vi "NIMS_NS_fir_lpnorm.vi"(5 "Function name":string, 6 "Line number":i32, 7 "Number of outputs requested":i32, 8 "error in (no error)":errorcluster, 11 "[A]":variant[](array[variant])) -> (0 "error out":errorcluster, 3 "[funct(A)]":variant[](array[variant]))   [LabVIEW 2017]
uses:
  <vilib>/imath/engines/lvmath/Functions/Error Handling/error.ctl
  <instcachedir>/0/NIMS_RunTimeType_From StrictType (excl LVString)_1019F277F0A747EDBCA0F6C52CA54500.lvgen/NIMS_RunTimeType_From StrictType (excl LVString)_1019F277F0A747EDBCA0F6C52CA54500_000.vi
  <instcachedir>/0/NIMS_Get Scalar_w Error_1987D997E87247DDAC16EA23A5E9E4FC.lvgen/NIMS_Get Scalar_w Error_1987D997E87247DDAC16EA23A5E9E4FC_000.vi
  <instcachedir>/0/NIMS_Complex To Real_BE01396FDE034E8E94CEBBA1E368668D.lvgen/NIMS_Complex To Real_BE01396FDE034E8E94CEBBA1E368668D_000.vi
  <instcachedir>/0/NIMS_Get Any Vector_w Error - Matrix_9FDB8FBE264C42EDBC8FF9BA66C3EF33.lvgen/NIMS_Get Any Vector_w Error - Matrix_9FDB8FBE264C42EDBC8FF9BA66C3EF33_001.vi
  <instcachedir>/0/NIMS_RunTimeType_To Numeric_1CBDAFC4EFAD4045A1DE52278D16738D.lvgen/NIMS_RunTimeType_To Numeric_1CBDAFC4EFAD4045A1DE52278D16738D_000.vi
  <vilib>/addons/Digital Filter Design/NI_DigFilter_MathScript.lvlib
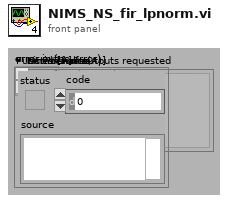
[diagram p1: front panel]
types:
  T1 = typedef "error.ctl" = enum16{"No Error", "Problem", "Input type must not be void", "Incorrect number of parameters", "Function not defined for non-numeric types", "An output variable of the user-defined function is undefined", "Function only defined for character arrays", "Function not defined for boolean, character, or single precision", "Function not defined for complex types", "Not a valid operation", "Inputs must be scalar", "Input matrices are not the same size", "Function only available on RT", "Input matrices must be nonnegative integers of the same type", "Arguments must be non-negative integers less than bitmax", "Number to complement must be less than 2^N", "Bit to get is outside range", "Bit to set is outside range", "Input must be real type ", "At least one parameter must be scalar", "Unable to display plug-in data on RT", "Function not defined for higher dimensional matrices", "Invalid attributes", "Wrong Type of Input Arguments", "Wrong Argument Option", "Invalid file identifier", "Indices must be real positive integers", "The variable is not a matrix data type.", "Number of elements must be the same for indices and values", "You cannot replace elements of a matrix with non-matrix data types.", "Cannot resize a 2D matrix with a linear index", "Unknown variable or symbol", "Indices out of range", "Empty matrix deletion can not be used with two indices", "Number of rows and columns must be the same for indices and values.", "Complex cannot be converted to Boolean", "Char cannot be converted to Boolean", "int64 cannot be converted to Boolean", "uint64 cannot be converted to Boolean", "You cannot convert a Boolean to a character.", "Incompatible input size in 3D surface function", "All rows must have the same number of columns", "Incompatible types", "Invalid matrix dimensions", "Dimension must be 1 or 2", "Base must be an integer between 2 and 36", "Invalid input", "Square matrix required", "Function 'timerstart' must be called before 'timerstop'", "Arguments must be positive real", "Step must not be zero", "Wrong number of input arguments", "Wrong number of output arguments", "Too many index arguments", "Input scalar must be >= 0", "Input scalar must be positive", "Input scalar must not be 0", "Input scalar must be in range [0,1]", "Can't use conditionally defined variable that's undefined", "Input must be a vector", "RT Exec Trace Toolkit not licensed", "Empty vector error", "All elements must be in domain [-1,1]", "All real elements of input vector must be >= 0", "All elements of input vector must be positive", "Values of input vectors are not compatible", "DAQmx not installed", "Input vector must be an increasing vector", "Dereferenced field does not exist within the struct", "A vector or matrix of structures must be indexed before it can be dereferenced", "Lenths of two input vectors are not compatible", "Invalid fieldname", "Empty matrix error", "Cannot use '.' on a type other than Struct", "Unused074", "Data type of the struct's field name is invalid", "Using . to dereference data that is not a struct", "Input struct contains invalid type ", "Size of input matrix is incompatible with input size", "Invalid format specifier", "Could not find field within struct", "Bad permutation array", "Mismatched fieldnames", "ode: User Function could not be opened", "ode: User Function signature does not meet ode requirements", "Unused085", "RunTime: MathScript could not be compiled", "Unknown function", "Only scalars and strings supported", "ode: User Function signature has incorrect number of inputs", "ode:User Function signature has incorrect number of outputs", "Range is too large", "End used without variable", "Function not available (RTE)", "Custom user error", "Arguments must be integers less than bitmax", "Shared library not found", "Header file not found", "Shared library already loaded", "Shared library not loaded", "Shared library function not found", "Shared library string return problem", "Problem calling shared library function", "Problem loading shared library from OS", "Problem parsing shared library header file", "Shared library incompatible types", "Shared library unsupported return type", "Shared library function not exported", "Shared library unsupported input type", "Problem unloading shared library from OS", "Function only available from UI", "Function specified in argument is missing", "An internal error has occurred", "Invalid object", "Invalid property", "Read-only property", "A break command has occurred", "A continue command has occurred", "A return command has occurred", "ode: times parameter invalid", "Function specified in argument has incorrect signature", "Function not found in file", "Reserved keyword cannot be defined as variable", "Reserved keyword cannot be defined as a function or script", "Arguments must be string literals", "Function not supported on this platform", "All columns must have the same number of rows", "Function ignored in RTE warning", "Cannot use : as a parameter that is not a variable", "Output can't be coerced to requested type", "Function not supported on current target", "Variable dependent on an unwired function input", "Unused132", "Unused133", "Unused134", "Unused135", "Unused136", "Unused137", "Unused138", "Unused139", "Global/Persistent must only take constants as arguments.", "Varargin must be last input in the function definition.", "Varargout must be last output in the function definition.", "Invalid output type. Cannot output a cell array of any type other than string.", "Invalid output type. Type is a dynamic struct.", "Invalid output type. Type is a struct that has a field whose type is not known until run-time", "Invalid output type. Type is a struct that has a field which is a plot object.", "MathScript parser DLL missing", "MathScript requires LabVIEW Full", "MathScript license is invalid or missing", "Varargout not supported except in assignments."}
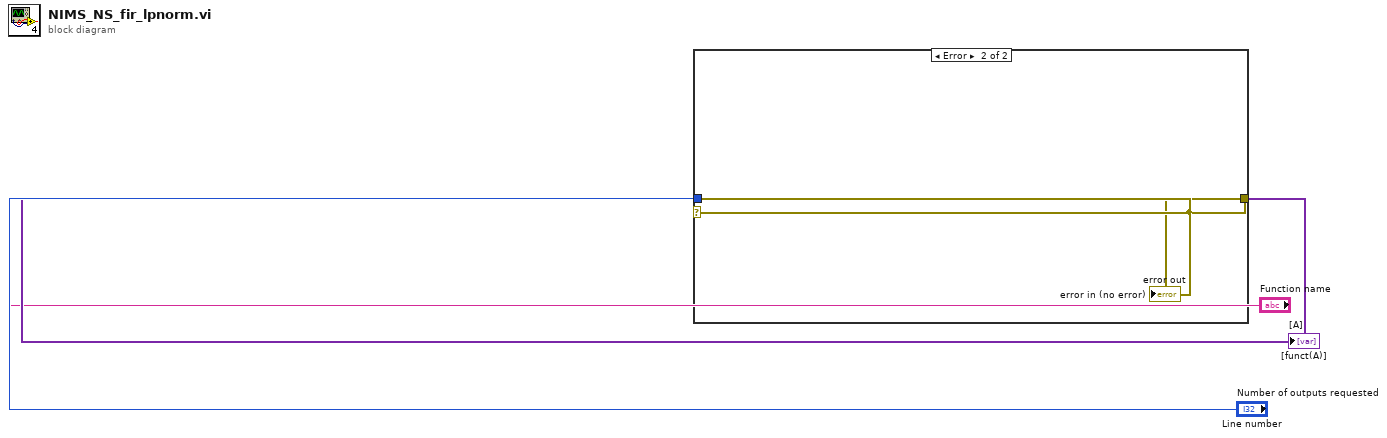
[diagram p0: block diagram]
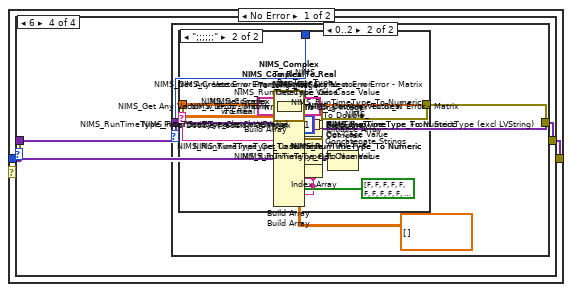
[diagram p2: hidden frame]
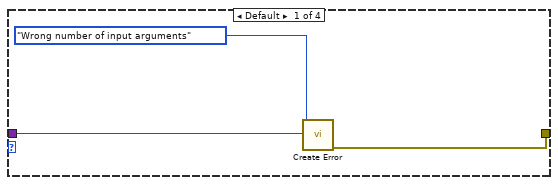
[diagram p3: hidden frame]
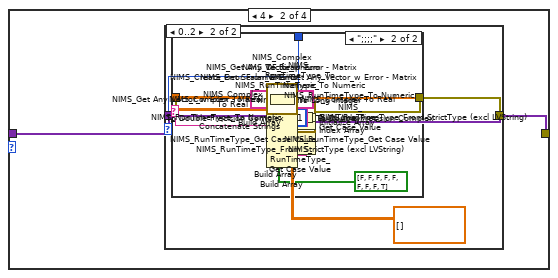
[diagram p4: hidden frame]
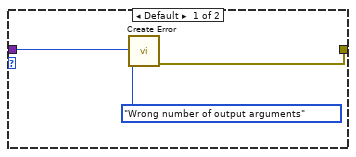
[diagram p5: hidden frame]
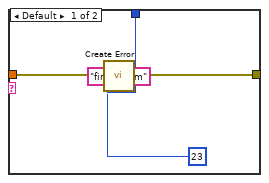
[diagram p6: hidden frame]
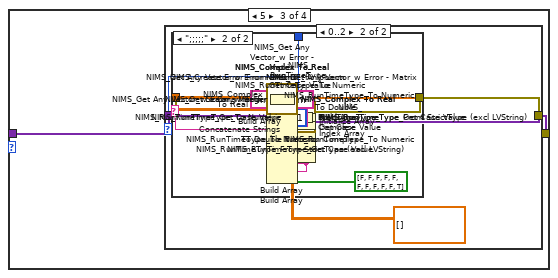
[diagram p7: hidden frame]
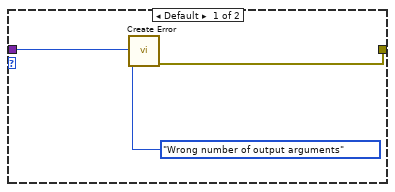
[diagram p8: hidden frame]
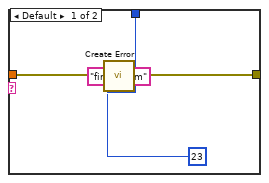
[diagram p9: hidden frame]
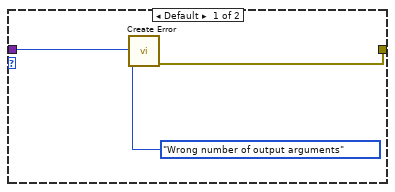
[diagram p10: hidden frame]
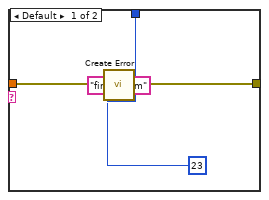
[diagram p11: hidden frame]
diagram:
  n1 = case shown="Error" "error in (no error)" {
    selector: "error in (no error)" -> [_ w295]
    tunnel: [w15 _] -> w4
    tunnel: [w14 w295] -> w3
    tunnel: "error in (no error)" -> [w13 _]
    tunnel: "Number of outputs requested" -> [w12 _]
    tunnel: "[A]" -> [w11 _]
    tunnel: "Function name" -> [w10 _]
    tunnel: "Line number" -> [w9 _]
    frame No Error {
      n2 = Array Size(array=w11) -> (size(s)=w8:i32)
      n3 = case shown="6" w8 {
        tunnel: [_ w27 w109 w200] -> w15
        tunnel: w10 -> [w19 w24 w106 w197]
        tunnel: w9 -> [w20 w25 w107 w198]
        tunnel: w13 -> [w17 w23 w105 w196]
        tunnel: [w16 w22 w104 w195] -> w14
        tunnel: w12 -> [_ w21 w103 w194]
        tunnel: w11 -> [_ w26 w108 w199]
        frame Default {
          n4 = call <vilib>:"Create Error.vi"("Function name"=w19, "error in (no error)"=w17, "Error Enum"=error."Wrong number of input arguments", "Line number"=w20) -> ("error out"=w16:errorcluster)  [unwired: 6 in, 1 out]
        }
        frame 4 {
          n5 = case shown="0..2" w21 {
            tunnel: [_ w33] -> w27
            tunnel: w24 -> [w31 _]
            tunnel: w25 -> [w32 w64]
            tunnel: w23 -> [w29 w62]
            tunnel: [w28 w45] -> w22
            tunnel: w26 -> [_ w65]
            frame Default {
              n6 = call <vilib>:"Create Error.vi"("Function name"=w31, "error in (no error)"=w29, "Error Enum"=error."Wrong number of output arguments", "Line number"=w32) -> ("error out"=w28:errorcluster)  [unwired: 6 in, 1 out]
            }
            frame 0..2 {
              w39 = 1
              n7 = Index Array(array=w65) -> (element #1=w61:variant, element #2=w57:variant, element #3=w53:variant, element #4=w49:variant)  [unwired: 4 in]
              n8 = call <vilib>:"NIMS_RunTimeType_Get Case Value.vi"("Data In"=w49) -> ("Case Value"=w46:string)  [unwired: 9 in, 1 out]
              n9 = call-generic <vilib>:"NIMS_RunTimeType_To Numeric.vi"("DataType"=cdb[][] [], "Variant"=w49) -> ("data"=w47:cdb[][])  [unwired: 1 in]
              n10 = call <vilib>:"NIMS_RunTimeType_Get Case Value.vi"("Data In"=w53) -> ("Case Value"=w50:string)  [unwired: 9 in, 1 out]
              n11 = call-generic <vilib>:"NIMS_RunTimeType_To Numeric.vi"("DataType"=cdb[][] [], "Variant"=w53) -> ("data"=w51:cdb[][])  [unwired: 1 in]
              n12 = call <vilib>:"NIMS_RunTimeType_Get Case Value.vi"("Data In"=w57) -> ("Case Value"=w54:string)  [unwired: 9 in, 1 out]
              n13 = call-generic <vilib>:"NIMS_RunTimeType_To Numeric.vi"("DataType"=cdb[][] [], "Variant"=w57) -> ("data"=w55:cdb[][])  [unwired: 1 in]
              n14 = call <vilib>:"NIMS_RunTimeType_Get Case Value.vi"("Data In"=w61) -> ("Case Value"=w58:string)  [unwired: 9 in, 1 out]
              n15 = call-generic <vilib>:"NIMS_RunTimeType_To Numeric.vi"("DataType"=cdb[][] [], "Variant"=w61) -> ("data"=w59:cdb[][])  [unwired: 1 in]
              n16 = Concatenate Strings(w58, w54, w50, w46) -> (w63:string)
              n17 = case shown="\";;;;\"" w63 {
                tunnel: w62 -> [w67 w77]
                tunnel: [_ w72] -> w44
                tunnel: [_ w71] -> w40
                tunnel: [w66 w73] -> w45
                tunnel: w59 -> [_ w101]
                tunnel: w55 -> [_ w97]
                tunnel: w51 -> [_ w94]
                tunnel: w47 -> [_ w91]
                tunnel: w64 -> [w70 w80]
                frame Default {
                  n18 = call <vilib>:"Create Error.vi"("Function name"="fir_lpnorm", "error in (no error)"=w67, "Error Enum"=23, "Line number"=w70) -> ("error out"=w66:errorcluster)  [unwired: 6 in, 1 out]
                }
                frame ";;;;" {
                  w75 = "fir_lpnorm"
                  n19 = call-generic <vilib>:"NIMS_Complex To Real.vi"("A"=w91) -> ("Error Enum"=w83:T1, "Real(A)"=w90:dbl[][])  [unwired: 8 in, 1 out]
                  n20 = call-generic <vilib>:"NIMS_Get Any Vector_w Error - Matrix.vi"("A"=w90) -> ("Error Enum"=w82:T1, "Vector"=w92:dbl[])  [unwired: 8 in, 1 out]
                  n21 = call-generic <vilib>:"NIMS_Complex To Real.vi"("A"=w94) -> ("Error Enum"=w85:T1, "Real(A)"=w93:dbl[][])  [unwired: 8 in, 1 out]
                  n22 = call-generic <vilib>:"NIMS_Get Any Vector_w Error - Matrix.vi"("A"=w93) -> ("Error Enum"=w84:T1, "Vector"=w95:dbl[])  [unwired: 8 in, 1 out]
                  n23 = call-generic <vilib>:"NIMS_Complex To Real.vi"("A"=w97) -> ("Error Enum"=w87:T1, "Real(A)"=w96:dbl[][])  [unwired: 8 in, 1 out]
                  n24 = call-generic <vilib>:"NIMS_Get Any Vector_w Error - Matrix.vi"("A"=w96) -> ("Error Enum"=w86:T1, "Vector"=w98:dbl[])  [unwired: 8 in, 1 out]
                  n25 = call-generic <vilib>:"NIMS_Complex To Real.vi"("A"=w101) -> ("Error Enum"=w89:T1, "Real(A)"=w100:dbl[][])  [unwired: 8 in, 1 out]
                  n26 = To Long Integer(number=w100) -> (32bit integer=w99:i32[][])
                  n27 = call-generic <vilib>:"NIMS_Get Scalar_w Error.vi"("A"=w99) -> ("Error Enum"=w88:T1, "Scalar"=w102:i32)  [unwired: 8 in, 1 out]
                  n28 = call <vilib>:"NIMS_DF_fir_lpnorm.vi"("mag"=w92, "e"=w95, "f"=w98, "n"=w102) -> ("error"=w81:i32, "err"=w71:dbl, "b"=w72:dbl[])  [unwired: 5 in]
                  n29 = Build Array(w75, w75, w75, w75, w75, w75, w75, w75, "fir_lpnorm") -> (w78:string[])
                  n30 = Build Array(w89, w88, w87, w86, w85, w84, w83, w82, w81) -> (w79:i32[])
                  n31 = call <vilib>:"NIMS_Create Error From Enums.vi"("Error Code"=bool[] [FALSE, FALSE, FALSE, FALSE, FALSE, FALSE, FALSE, FALSE, TRUE], "error in (no error)"=w77, "Line no"=w80, "Error Enums"=w79, "Function names"=w78) -> ("error out"=w73:errorcluster)  [unwired: 6 in]
                }
              }
              n32 = Initialize Array(w40, w39, w39) -> (w38:dbl[][])
              n33 = To Double Precision Complex(1:w38) -> (0:w37:cdb[][])
              n34 = call-generic <vilib>:"NIMS_RunTimeType_From StrictType (excl LVString).vi"("Plug-In Name"="", "Data In"=w37) -> ("Data Out"=w34:variant)  [unwired: 2 in]
              n35 = Build Array(w44) -> (w43:dbl[][])
              n36 = To Double Precision Complex(1:w43) -> (0:w42:cdb[][])
              n37 = call-generic <vilib>:"NIMS_RunTimeType_From StrictType (excl LVString).vi"("Plug-In Name"="", "Data In"=w42) -> ("Data Out"=w35:variant)  [unwired: 2 in]
              n38 = Build Array(w35, w34) -> (w33:variant[])
            }
          }
        }
        frame 5 {
          n39 = case shown="0..2" w103 {
            tunnel: [_ w115] -> w109
            tunnel: w106 -> [w113 _]
            tunnel: w107 -> [w114 w150]
            tunnel: w105 -> [w111 w148]
            tunnel: [w110 w127] -> w104
            tunnel: w108 -> [_ w151]
            frame Default {
              n40 = call <vilib>:"Create Error.vi"("Function name"=w113, "error in (no error)"=w111, "Error Enum"=error."Wrong number of output arguments", "Line number"=w114) -> ("error out"=w110:errorcluster)  [unwired: 6 in, 1 out]
            }
            frame 0..2 {
              w121 = 1
              n41 = Index Array(array=w151) -> (element #1=w147:variant, element #2=w143:variant, element #3=w139:variant, element #4=w135:variant, element #5=w131:variant)  [unwired: 5 in]
              n42 = call <vilib>:"NIMS_RunTimeType_Get Case Value.vi"("Data In"=w131) -> ("Case Value"=w128:string)  [unwired: 9 in, 1 out]
              n43 = call-generic <vilib>:"NIMS_RunTimeType_To Numeric.vi"("DataType"=cdb[][] [], "Variant"=w131) -> ("data"=w129:cdb[][])  [unwired: 1 in]
              n44 = call <vilib>:"NIMS_RunTimeType_Get Case Value.vi"("Data In"=w135) -> ("Case Value"=w132:string)  [unwired: 9 in, 1 out]
              n45 = call-generic <vilib>:"NIMS_RunTimeType_To Numeric.vi"("DataType"=cdb[][] [], "Variant"=w135) -> ("data"=w133:cdb[][])  [unwired: 1 in]
              n46 = call <vilib>:"NIMS_RunTimeType_Get Case Value.vi"("Data In"=w139) -> ("Case Value"=w136:string)  [unwired: 9 in, 1 out]
              n47 = call-generic <vilib>:"NIMS_RunTimeType_To Numeric.vi"("DataType"=cdb[][] [], "Variant"=w139) -> ("data"=w137:cdb[][])  [unwired: 1 in]
              n48 = call <vilib>:"NIMS_RunTimeType_Get Case Value.vi"("Data In"=w143) -> ("Case Value"=w140:string)  [unwired: 9 in, 1 out]
              n49 = call-generic <vilib>:"NIMS_RunTimeType_To Numeric.vi"("DataType"=cdb[][] [], "Variant"=w143) -> ("data"=w141:cdb[][])  [unwired: 1 in]
              n50 = call <vilib>:"NIMS_RunTimeType_Get Case Value.vi"("Data In"=w147) -> ("Case Value"=w144:string)  [unwired: 9 in, 1 out]
              n51 = call-generic <vilib>:"NIMS_RunTimeType_To Numeric.vi"("DataType"=cdb[][] [], "Variant"=w147) -> ("data"=w145:cdb[][])  [unwired: 1 in]
              n52 = Concatenate Strings(w144, w140, w136, w132, w128) -> (w149:string)
              n53 = case shown="\";;;;;\"" w149 {
                tunnel: w148 -> [w153 w163]
                tunnel: [_ w158] -> w126
                tunnel: [_ w157] -> w122
                tunnel: [w152 w159] -> w127
                tunnel: w145 -> [_ w192]
                tunnel: w141 -> [_ w188]
                tunnel: w137 -> [_ w185]
                tunnel: w133 -> [_ w182]
                tunnel: w129 -> [_ w179]
                tunnel: w150 -> [w156 w166]
                frame Default {
                  n54 = call <vilib>:"Create Error.vi"("Function name"="fir_lpnorm", "error in (no error)"=w153, "Error Enum"=23, "Line number"=w156) -> ("error out"=w152:errorcluster)  [unwired: 6 in, 1 out]
                }
                frame ";;;;;" {
                  w161 = "fir_lpnorm"
                  n55 = call-generic <vilib>:"NIMS_Complex To Real.vi"("A"=w179) -> ("Error Enum"=w169:T1, "Real(A)"=w178:dbl[][])  [unwired: 8 in, 1 out]
                  n56 = call-generic <vilib>:"NIMS_Get Any Vector_w Error - Matrix.vi"("A"=w178) -> ("Error Enum"=w168:T1, "Vector"=w180:dbl[])  [unwired: 8 in, 1 out]
                  n57 = call-generic <vilib>:"NIMS_Complex To Real.vi"("A"=w182) -> ("Error Enum"=w171:T1, "Real(A)"=w181:dbl[][])  [unwired: 8 in, 1 out]
                  n58 = call-generic <vilib>:"NIMS_Get Any Vector_w Error - Matrix.vi"("A"=w181) -> ("Error Enum"=w170:T1, "Vector"=w183:dbl[])  [unwired: 8 in, 1 out]
                  n59 = call-generic <vilib>:"NIMS_Complex To Real.vi"("A"=w185) -> ("Error Enum"=w173:T1, "Real(A)"=w184:dbl[][])  [unwired: 8 in, 1 out]
                  n60 = call-generic <vilib>:"NIMS_Get Any Vector_w Error - Matrix.vi"("A"=w184) -> ("Error Enum"=w172:T1, "Vector"=w186:dbl[])  [unwired: 8 in, 1 out]
                  n61 = call-generic <vilib>:"NIMS_Complex To Real.vi"("A"=w188) -> ("Error Enum"=w175:T1, "Real(A)"=w187:dbl[][])  [unwired: 8 in, 1 out]
                  n62 = call-generic <vilib>:"NIMS_Get Any Vector_w Error - Matrix.vi"("A"=w187) -> ("Error Enum"=w174:T1, "Vector"=w189:dbl[])  [unwired: 8 in, 1 out]
                  n63 = call-generic <vilib>:"NIMS_Complex To Real.vi"("A"=w192) -> ("Error Enum"=w177:T1, "Real(A)"=w191:dbl[][])  [unwired: 8 in, 1 out]
                  n64 = To Long Integer(number=w191) -> (32bit integer=w190:i32[][])
                  n65 = call-generic <vilib>:"NIMS_Get Scalar_w Error.vi"("A"=w190) -> ("Error Enum"=w176:T1, "Scalar"=w193:i32)  [unwired: 8 in, 1 out]
                  n66 = call <vilib>:"NIMS_DF_fir_lpnorm.vi"("w"=w180, "mag"=w183, "e"=w186, "f"=w189, "n"=w193) -> ("error"=w167:i32, "err"=w157:dbl, "b"=w158:dbl[])  [unwired: 4 in]
                  n67 = Build Array(w161, w161, w161, w161, w161, w161, w161, w161, w161, w161, "fir_lpnorm") -> (w164:string[])
                  n68 = Build Array(w177, w176, w175, w174, w173, w172, w171, w170, w169, w168, w167) -> (w165:i32[])
                  n69 = call <vilib>:"NIMS_Create Error From Enums.vi"("Error Code"=bool[] [FALSE, FALSE, FALSE, FALSE, FALSE, FALSE, FALSE, FALSE, FALSE, FALSE, TRUE], "error in (no error)"=w163, "Line no"=w166, "Error Enums"=w165, "Function names"=w164) -> ("error out"=w159:errorcluster)  [unwired: 6 in]
                }
              }
              n70 = Initialize Array(w122, w121, w121) -> (w120:dbl[][])
              n71 = To Double Precision Complex(1:w120) -> (0:w119:cdb[][])
              n72 = call-generic <vilib>:"NIMS_RunTimeType_From StrictType (excl LVString).vi"("Plug-In Name"="", "Data In"=w119) -> ("Data Out"=w116:variant)  [unwired: 2 in]
              n73 = Build Array(w126) -> (w125:dbl[][])
              n74 = To Double Precision Complex(1:w125) -> (0:w124:cdb[][])
              n75 = call-generic <vilib>:"NIMS_RunTimeType_From StrictType (excl LVString).vi"("Plug-In Name"="", "Data In"=w124) -> ("Data Out"=w117:variant)  [unwired: 2 in]
              n76 = Build Array(w117, w116) -> (w115:variant[])
            }
          }
        }
        frame 6 {
          n77 = case shown="0..2" w194 {
            tunnel: [_ w206] -> w200
            tunnel: w197 -> [w204 _]
            tunnel: w198 -> [w205 w245]
            tunnel: w196 -> [w202 w243]
            tunnel: [w201 w218] -> w195
            tunnel: w199 -> [_ w246]
            frame Default {
              n78 = call <vilib>:"Create Error.vi"("Function name"=w204, "error in (no error)"=w202, "Error Enum"=error."Wrong number of output arguments", "Line number"=w205) -> ("error out"=w201:errorcluster)  [unwired: 6 in, 1 out]
            }
            frame 0..2 {
              w212 = 1
              n79 = Index Array(array=w246) -> (element #1=w242:variant, element #2=w238:variant, element #3=w234:variant, element #4=w230:variant, element #5=w226:variant, element #6=w222:variant)  [unwired: 6 in]
              n80 = call <vilib>:"NIMS_RunTimeType_Get Case Value.vi"("Data In"=w222) -> ("Case Value"=w219:string)  [unwired: 9 in, 1 out]
              n81 = call-generic <vilib>:"NIMS_RunTimeType_To Numeric.vi"("DataType"=cdb[][] [], "Variant"=w222) -> ("data"=w220:cdb[][])  [unwired: 1 in]
              n82 = call <vilib>:"NIMS_RunTimeType_Get Case Value.vi"("Data In"=w226) -> ("Case Value"=w223:string)  [unwired: 9 in, 1 out]
              n83 = call-generic <vilib>:"NIMS_RunTimeType_To Numeric.vi"("DataType"=cdb[][] [], "Variant"=w226) -> ("data"=w224:cdb[][])  [unwired: 1 in]
              n84 = call <vilib>:"NIMS_RunTimeType_Get Case Value.vi"("Data In"=w230) -> ("Case Value"=w227:string)  [unwired: 9 in, 1 out]
              n85 = call-generic <vilib>:"NIMS_RunTimeType_To Numeric.vi"("DataType"=cdb[][] [], "Variant"=w230) -> ("data"=w228:cdb[][])  [unwired: 1 in]
              n86 = call <vilib>:"NIMS_RunTimeType_Get Case Value.vi"("Data In"=w234) -> ("Case Value"=w231:string)  [unwired: 9 in, 1 out]
              n87 = call-generic <vilib>:"NIMS_RunTimeType_To Numeric.vi"("DataType"=cdb[][] [], "Variant"=w234) -> ("data"=w232:cdb[][])  [unwired: 1 in]
              n88 = call <vilib>:"NIMS_RunTimeType_Get Case Value.vi"("Data In"=w238) -> ("Case Value"=w235:string)  [unwired: 9 in, 1 out]
              n89 = call-generic <vilib>:"NIMS_RunTimeType_To Numeric.vi"("DataType"=cdb[][] [], "Variant"=w238) -> ("data"=w236:cdb[][])  [unwired: 1 in]
              n90 = call <vilib>:"NIMS_RunTimeType_Get Case Value.vi"("Data In"=w242) -> ("Case Value"=w239:string)  [unwired: 9 in, 1 out]
              n91 = call-generic <vilib>:"NIMS_RunTimeType_To Numeric.vi"("DataType"=cdb[][] [], "Variant"=w242) -> ("data"=w240:cdb[][])  [unwired: 1 in]
              n92 = Concatenate Strings(w239, w235, w231, w227, w223, w219) -> (w244:string)
              n93 = case shown="\";;;;;;\"" w244 {
                tunnel: w243 -> [w248 w258]
                tunnel: [_ w253] -> w217
                tunnel: [_ w252] -> w213
                tunnel: [w247 w254] -> w218
                tunnel: w240 -> [_ w293]
                tunnel: w236 -> [_ w289]
                tunnel: w232 -> [_ w286]
                tunnel: w228 -> [_ w283]
                tunnel: w224 -> [_ w280]
                tunnel: w220 -> [_ w277]
                tunnel: w245 -> [w251 w261]
                frame Default {
                  n94 = call <vilib>:"Create Error.vi"("Function name"="fir_lpnorm", "error in (no error)"=w248, "Error Enum"=23, "Line number"=w251) -> ("error out"=w247:errorcluster)  [unwired: 6 in, 1 out]
                }
                frame ";;;;;;" {
                  w256 = "fir_lpnorm"
                  n95 = call-generic <vilib>:"NIMS_Complex To Real.vi"("A"=w277) -> ("Error Enum"=w264:T1, "Real(A)"=w276:dbl[][])  [unwired: 8 in, 1 out]
                  n96 = To Long Integer(number=w276) -> (32bit integer=w275:i32[][])
                  n97 = call-generic <vilib>:"NIMS_Get Scalar_w Error.vi"("A"=w275) -> ("Error Enum"=w263:T1, "Scalar"=w278:i32)  [unwired: 8 in, 1 out]
                  n98 = call-generic <vilib>:"NIMS_Complex To Real.vi"("A"=w280) -> ("Error Enum"=w266:T1, "Real(A)"=w279:dbl[][])  [unwired: 8 in, 1 out]
                  n99 = call-generic <vilib>:"NIMS_Get Any Vector_w Error - Matrix.vi"("A"=w279) -> ("Error Enum"=w265:T1, "Vector"=w281:dbl[])  [unwired: 8 in, 1 out]
                  n100 = call-generic <vilib>:"NIMS_Complex To Real.vi"("A"=w283) -> ("Error Enum"=w268:T1, "Real(A)"=w282:dbl[][])  [unwired: 8 in, 1 out]
                  n101 = call-generic <vilib>:"NIMS_Get Any Vector_w Error - Matrix.vi"("A"=w282) -> ("Error Enum"=w267:T1, "Vector"=w284:dbl[])  [unwired: 8 in, 1 out]
                  n102 = call-generic <vilib>:"NIMS_Complex To Real.vi"("A"=w286) -> ("Error Enum"=w270:T1, "Real(A)"=w285:dbl[][])  [unwired: 8 in, 1 out]
                  n103 = call-generic <vilib>:"NIMS_Get Any Vector_w Error - Matrix.vi"("A"=w285) -> ("Error Enum"=w269:T1, "Vector"=w287:dbl[])  [unwired: 8 in, 1 out]
                  n104 = call-generic <vilib>:"NIMS_Complex To Real.vi"("A"=w289) -> ("Error Enum"=w272:T1, "Real(A)"=w288:dbl[][])  [unwired: 8 in, 1 out]
                  n105 = call-generic <vilib>:"NIMS_Get Any Vector_w Error - Matrix.vi"("A"=w288) -> ("Error Enum"=w271:T1, "Vector"=w290:dbl[])  [unwired: 8 in, 1 out]
                  n106 = call-generic <vilib>:"NIMS_Complex To Real.vi"("A"=w293) -> ("Error Enum"=w274:T1, "Real(A)"=w292:dbl[][])  [unwired: 8 in, 1 out]
                  n107 = To Long Integer(number=w292) -> (32bit integer=w291:i32[][])
                  n108 = call-generic <vilib>:"NIMS_Get Scalar_w Error.vi"("A"=w291) -> ("Error Enum"=w273:T1, "Scalar"=w294:i32)  [unwired: 8 in, 1 out]
                  n109 = call <vilib>:"NIMS_DF_fir_lpnorm.vi"("p"=w278, "w"=w281, "mag"=w284, "e"=w287, "f"=w290, "n"=w294) -> ("error"=w262:i32, "err"=w252:dbl, "b"=w253:dbl[])  [unwired: 3 in]
                  n110 = Build Array(w256, w256, w256, w256, w256, w256, w256, w256, w256, w256, w256, w256, "fir_lpnorm") -> (w259:string[])
                  n111 = Build Array(w274, w273, w272, w271, w270, w269, w268, w267, w266, w265, w264, w263, w262) -> (w260:i32[])
                  n112 = call <vilib>:"NIMS_Create Error From Enums.vi"("Error Code"=bool[] [FALSE, FALSE, FALSE, FALSE, FALSE, FALSE, FALSE, FALSE, FALSE, FALSE, FALSE, FALSE, TRUE], "error in (no error)"=w258, "Line no"=w261, "Error Enums"=w260, "Function names"=w259) -> ("error out"=w254:errorcluster)  [unwired: 6 in]
                }
              }
              n113 = Initialize Array(w213, w212, w212) -> (w211:dbl[][])
              n114 = To Double Precision Complex(1:w211) -> (0:w210:cdb[][])
              n115 = call-generic <vilib>:"NIMS_RunTimeType_From StrictType (excl LVString).vi"("Plug-In Name"="", "Data In"=w210) -> ("Data Out"=w207:variant)  [unwired: 2 in]
              n116 = Build Array(w217) -> (w216:dbl[][])
              n117 = To Double Precision Complex(1:w216) -> (0:w215:cdb[][])
              n118 = call-generic <vilib>:"NIMS_RunTimeType_From StrictType (excl LVString).vi"("Plug-In Name"="", "Data In"=w215) -> ("Data Out"=w208:variant)  [unwired: 2 in]
              n119 = Build Array(w208, w207) -> (w206:variant[])
            }
          }
        }
      }
    }
    frame Error {
    }
  }
  "error out" <- w3
  "[funct(A)]" <- w4
